vi "Connect Verify.vi"(8 "error in (no error)":errorcluster, 10 "Targets in":T1 {"Filtered Targets"."IP Mode" items=["Static"=1, "DHCP/Link-Local"=2, "Link-Local Only"=4, "DHCP Only"=8]}, 11 "Ctl Refs":T6) -> (0 "error out":errorcluster, 2 "Button state":T5, 3 "Execution state":T4)   [LabVIEW 2013]
uses:
  Controls/Refs.ctl
  Controls/Button Refs.ctl
  Controls/Tab Ctl Refs.ctl
  types/TabStateType.ctl
  Controls/Indicator Refs.ctl
  Controls/Slider Refs.ctl
  Controls/Control Refs.ctl
  types/ButtonStateType.ctl
  types/ExecutionStateType.ctl
  Controls/Targets.ctl
  Controls/Detected.ctl
  types/MAX Sys Cfg Target Information.ctl
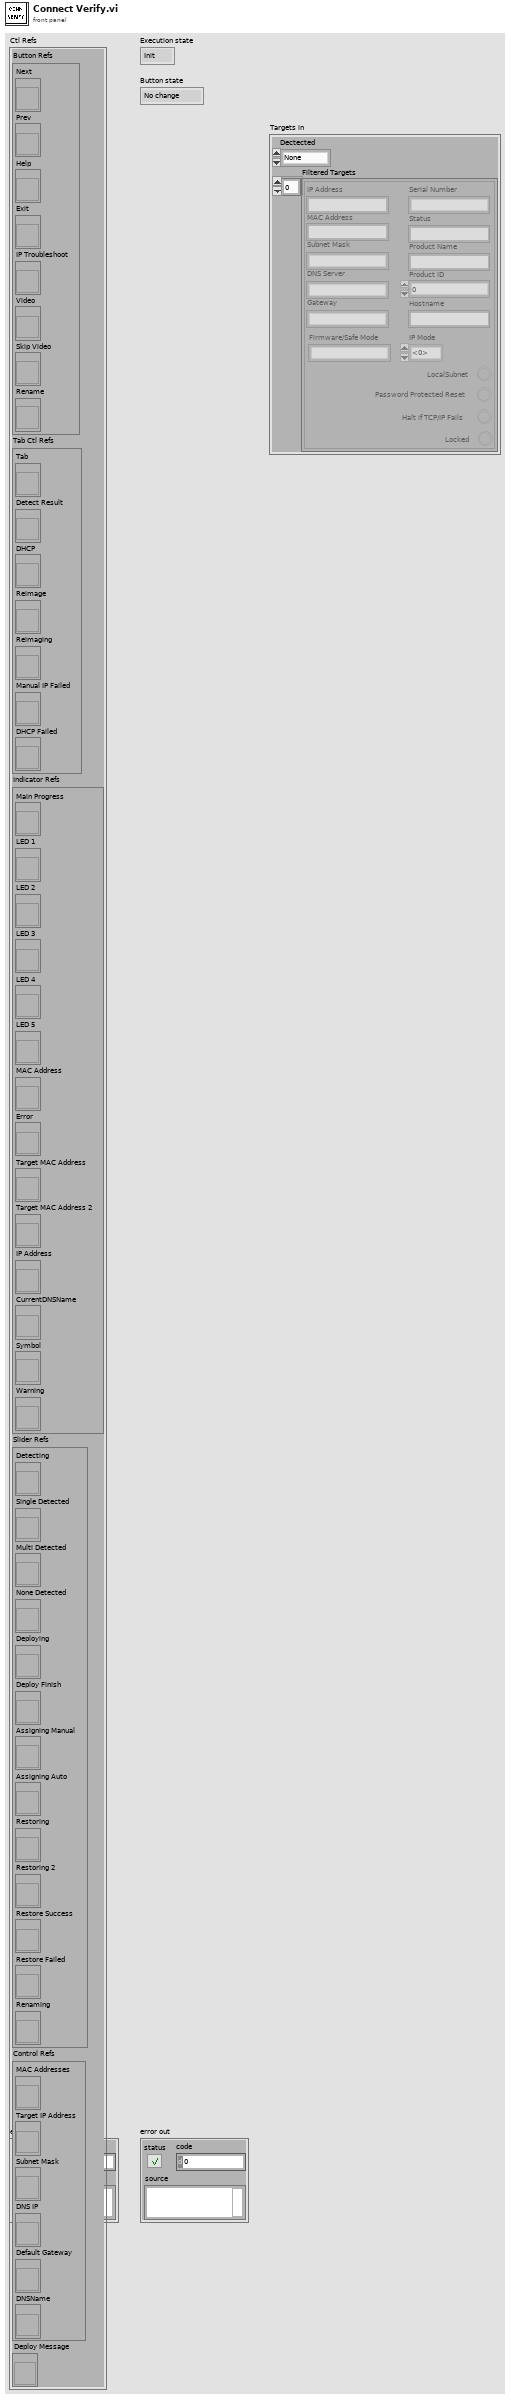
[diagram p1: front panel]
types:
  T1 = typedef "Targets.ctl" = cluster{"Dectected":T2, "Filtered Targets":T3[]}
  T2 = typedef "Detected.ctl" = enum16{"None", "Failed", "Single", "Multi"}
  T3 = typedef "MAX Sys Cfg Target Information.ctl" = cluster{"MAC Address":string, "IP Address":string, "Status":string, "Product Name":string, "Hostname":string, "Firmware/Safe Mode":string, "Subnet Mask":string, "Gateway":string, "DNS Server":string, "Serial Number":string, "Product ID":u32, "Locked ":bool, "LocalSubnet":bool, "Halt If TCP/IP Fails":bool, "Password Protected Reset":bool, "IP Mode":i32}
  T4 = typedef "ExecutionStateType.ctl" = enum16{"Init", "Welcome", "Idle", "Detect", "Run Detection", "Detect Fail", "Detect One", "Detect Mult", "Deploy", "DHCP", "Static IP", "Run Deployment", "Connect Verify", "Exit", "Video Wait", "Success", "Troubleshoot", "Troubleshoot 2", "RenameDNS"}
  T5 = typedef "ButtonStateType.ctl" = enum16{"No change", "No Next", "No Prev", "All Disabled", "All Enabled", "Exit Only"}
  T6 = typedef "Refs.ctl" = cluster{"Button Refs":T7, "Tab Ctl Refs":T8, "Indicator Refs":T9, "Slider Refs":T10, "Control Refs":T11, "Deploy Message":refnum<vi>}
  T7 = typedef "Button Refs.ctl" = cluster{"Next":refnum<vi>, "Prev":refnum<vi>, "Help":refnum<vi>, "Exit":refnum<vi>, "IP Troubleshoot":refnum<vi>, "Video":refnum<vi>, "Skip Video":refnum<vi>, "Rename":refnum<vi>}
  T8 = typedef "Tab Ctl Refs.ctl" = cluster{"Tab":refnum<vi>, "Detect Result":refnum<vi>, "DHCP":refnum<vi>, "Reimage":refnum<vi>, "Reimaging":refnum<vi>, "Manual IP Failed":refnum<vi>, "DHCP Failed":refnum<vi>}
  T9 = typedef "Indicator Refs.ctl" = cluster{"Main Progress":refnum<vi>, "LED 1":refnum<vi>, "LED 2":refnum<vi>, "LED 3":refnum<vi>, "LED 4":refnum<vi>, "LED 5":refnum<vi>, "MAC Address":refnum<vi>, "Error":refnum<vi>, "Target MAC Address":refnum<vi>, "Target MAC Address 2":refnum<vi>, "IP Address":refnum<vi>, "CurrentDNSName":refnum<vi>, "Symbol":refnum<vi>, "Warning":refnum<vi>}
  T10 = typedef "Slider Refs.ctl" = cluster{"Detecting":refnum<vi>, "Single Detected":refnum<vi>, "Multi Detected":refnum<vi>, "None Detected":refnum<vi>, "Deploying":refnum<vi>, "Deploy Finish":refnum<vi>, "Assigning Manual":refnum<vi>, "Assigning Auto":refnum<vi>, "Restoring":refnum<vi>, "Restoring 2":refnum<vi>, "Restore Success":refnum<vi>, "Restore Failed":refnum<vi>, "Renaming":refnum<vi>}
  T11 = typedef "Control Refs.ctl" = cluster{"MAC Addresses":refnum<vi>, "Target IP Address":refnum<vi>, "Subnet Mask":refnum<vi>, "DNS IP":refnum<vi>, "Default Gateway":refnum<vi>, "DNSName":refnum<vi>}
  T12 = enum8{"Enabled", "Disabled", "Disabled and Grayed Out"}
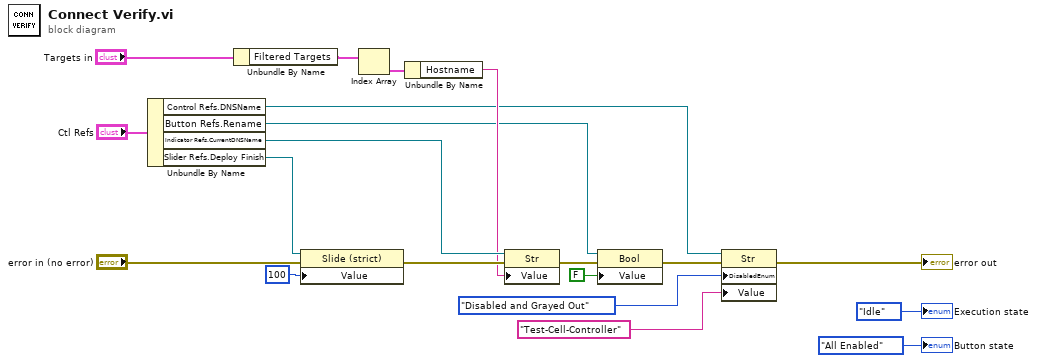
[diagram p0: block diagram]
diagram:
  n1 = Unbundle By Name("Ctl Refs") -> ("Control Refs.DNSName"=w3:refnum<vi>, "Button Refs.Rename"=w6:refnum<vi>, "Indicator Refs.CurrentDNSName"=w10:refnum<vi>, "Slider Refs.Deploy Finish"=w19:refnum<vi>)
  n2 = Unbundle By Name("Targets in") -> ("Filtered Targets"=w13:T3[])
  n3 = property on="Property Node" class="Slide (strict)"(reference=w19, error in="error in (no error)", "Value"=i8 100 ("Slide 3")) -> (error out=w11:errorcluster)  [unwired: 1 out]
  n4 = Index Array(array=w13) -> (element=w12:T3)  [unwired: 1 in]
  n5 = Unbundle By Name(w12) -> ("Hostname"=w9:string)
  n6 = property on="Property Node" class="Str"(reference=w10, error in=w11, "Value"=w9) -> (error out=w8:errorcluster)  [unwired: 1 out]
  n7 = property class="Bool"(reference=w6, error in=w8, "Value"=FALSE) -> (error out=w7:errorcluster)  [unwired: 1 out]
  n8 = property class="Str"(reference=w3, error in=w7, "DisabledEnum"=T12."Disabled and Grayed Out" ("Disabled"), "Value"="Test-Cell-Controller") -> (error out=→"error out":errorcluster)  [unwired: 1 out]
  "Button state" <- ButtonStateType."All Enabled" ("Enum")
  "Execution state" <- ExecutionStateType."Idle" ("Enum")
